vi "整線小幫手.vi"() -> ()   [LabVIEW 2015]
panel:
  in  "error in":errorcluster
  out "error out":errorcluster
  out "Refnum out":refnum<vi>
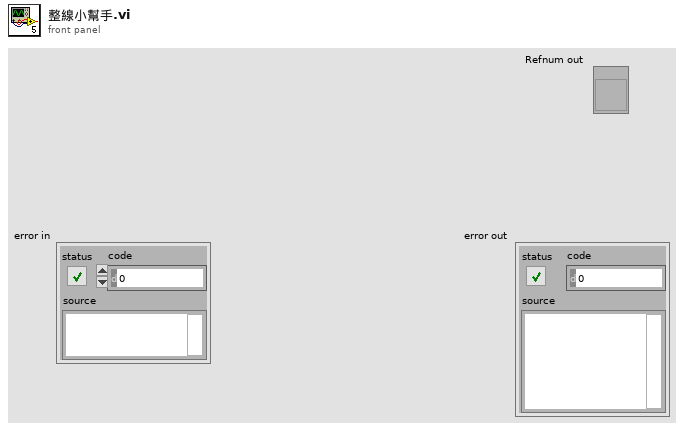
[diagram p1: front panel]
types:
  T1 = typedef "LVPositionTypeDef.ctl" = cluster{"Left":i32, "Top":i32}
  T2 = typedef "LVBoundsTypeDef.ctl" = cluster{"Width":u32, "Height":u32}
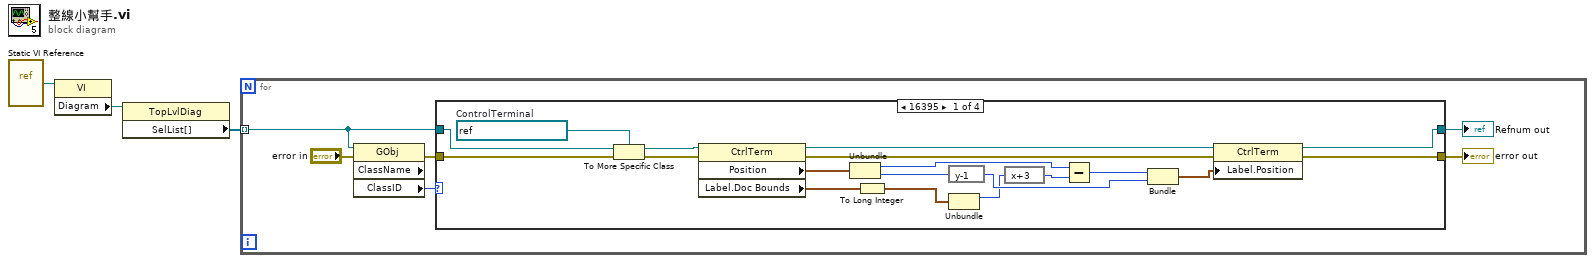
[diagram p0: block diagram]
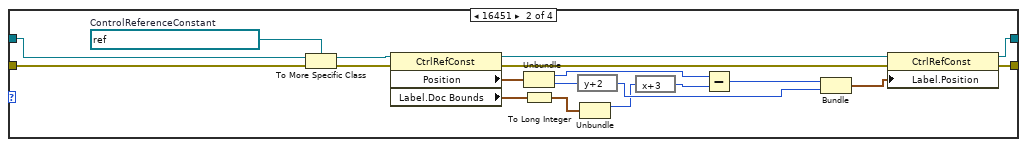
[diagram p2: hidden frame]
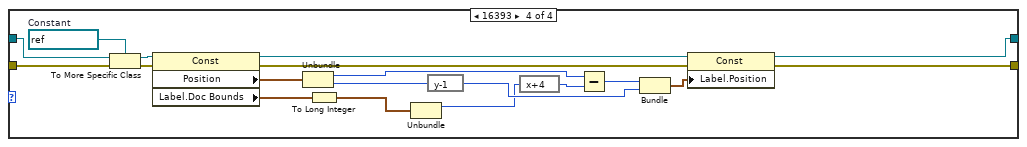
[diagram p4: hidden frame]
diagram:
  n1 = vi-ref "Static VI Reference"() -> ("vi reference"=w1:refnum<vi>)
  n2 = property on="Property Node" class="VI"(reference=w1) -> ("Diagram"=w3:refnum<vi>)  [unwired: 1 in, 2 out]
  n3 = property on="Property Node" class="TopLvlDiag"(reference=w3) -> ("SelList[]"=w2:refnum<vi>[])  [unwired: 1 in, 2 out]
  n4 = for {
    tunnel: w2 -> [w4] mode=indexing
    n5 = property on="Property Node" class="GObj" props=["ClassName", "ClassID"](reference=w4, error in="error in") -> (error out=w6:errorcluster, "ClassID"=w7:u32)  [unwired: 2 out]
    n6 = case shown="16395" w7 {
      tunnel: w6 -> [w14 w47 w48 w52]
      tunnel: w4 -> [w15 w46 w49 w53]
      tunnel: [w13 w45 w49 w51] -> w8
      tunnel: [w12 w44 w48 w50] -> w9
      frame 16395 {
        w28 = refnum<vi> refnum  # ControlTerminal
        n7 = To More Specific Class(target class=w28, reference=w15, error in=w14) -> (specific class reference=w11:refnum<vi>, error out=w10:errorcluster)
        n8 = property on="Property Node" class="CtrlTerm"(reference=w11, error in=w10) -> (reference out=w27:refnum<vi>, error out=w18:errorcluster, "Position"=w26:T1, "Label.Doc Bounds"=w17:T2)
        n9 = Unbundle(w26) -> ("Left"=w21:i32, "Top"=w23:i32)
        n10 = To Long Integer(number=w17) -> (32bit integer=w16:cluster{"Width":i32, "Height":i32})
        n11 = expression code="y-1"(w23) -> (w24:i32)
        n12 = Unbundle(w16) -> ("Width"=w22:i32)  [unwired: 1 out]
        n13 = expression code="x+3"(w22) -> (w20:i32)
        n14 = Subtract(x=w21, y=w20) -> (x-y=w19:i32)
        n15 = Bundle(w19, "Top"=w24) -> (w25:cluster{i32, "Top":i32})  [unwired: 1 in]
        n16 = property on="Property Node" class="CtrlTerm"(reference=w27, error in=w18, "Label.Position"=w25) -> (reference out=w13:refnum<vi>, error out=w12:errorcluster)
      }
      frame 16451 {
        w43 = refnum<vi> refnum  # ControlReferenceConstant
        n17 = To More Specific Class(target class=w43, reference=w46, error in=w47) -> (specific class reference=w42:refnum<vi>, error out=w41:errorcluster)
        n18 = property on="Property Node" class="CtrlRefConst"(reference=w42, error in=w41) -> (reference out=w40:refnum<vi>, error out=w31:errorcluster, "Position"=w39:T1, "Label.Doc Bounds"=w30:T2)
        n19 = Unbundle(w39) -> ("Left"=w34:i32, "Top"=w36:i32)
        n20 = To Long Integer(number=w30) -> (32bit integer=w29:cluster{"Width":i32, "Height":i32})
        n21 = expression code="y+2"(w36) -> (w37:i32)
        n22 = Unbundle(w29) -> ("Width"=w35:i32)  [unwired: 1 out]
        n23 = expression code="x+3"(w35) -> (w33:i32)
        n24 = Subtract(x=w34, y=w33) -> (x-y=w32:i32)
        n25 = Bundle(w32, "Top"=w37) -> (w38:cluster{i32, "Top":i32})  [unwired: 1 in]
        n26 = property on="Property Node" class="CtrlRefConst"(reference=w40, error in=w31, "Label.Position"=w38) -> (reference out=w45:refnum<vi>, error out=w44:errorcluster)
      }
      frame Default {
      }
      frame 16393 {
        w68 = refnum<vi> refnum  # Constant
        n27 = To More Specific Class(target class=w68, reference=w53, error in=w52) -> (specific class reference=w67:refnum<vi>, error out=w66:errorcluster)
        n28 = property on="Property Node" class="Const"(reference=w67, error in=w66) -> (reference out=w65:refnum<vi>, error out=w56:errorcluster, "Position"=w64:T1, "Label.Doc Bounds"=w55:T2)
        n29 = Unbundle(w64) -> ("Left"=w59:i32, "Top"=w61:i32)
        n30 = To Long Integer(number=w55) -> (32bit integer=w54:cluster{"Width":i32, "Height":i32})
        n31 = Unbundle(w54) -> ("Width"=w60:i32)  [unwired: 1 out]
        n32 = expression code="y-1"(w61) -> (w62:i32)
        n33 = expression code="x+4"(w60) -> (w58:i32)
        n34 = Subtract(x=w59, y=w58) -> (x-y=w57:i32)
        n35 = Bundle(w57, "Top"=w62) -> (w63:cluster{i32, "Top":i32})  [unwired: 1 in]
        n36 = property on="Property Node" class="Const"(reference=w65, error in=w56, "Label.Position"=w63) -> (reference out=w51:refnum<vi>, error out=w50:errorcluster)
      }
    }
    "error out" <- w9
    "Refnum out" <- w8
  }
